vi "tmp-valveControl.vi"() -> ()   [LabVIEW 2016]
uses:
  Classes/Controllers/I-O/Copy of NI-DAQ Folder/NI-DAQ.lvclass
panel:
  in  "values":bool[](array[boolean])=[TRUE]
  in  "indices":i32[](array[numeric])=[0]
  in  "DAQ Module":i32
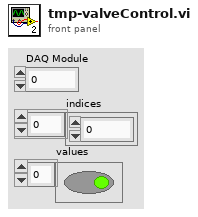
[diagram p1: front panel]
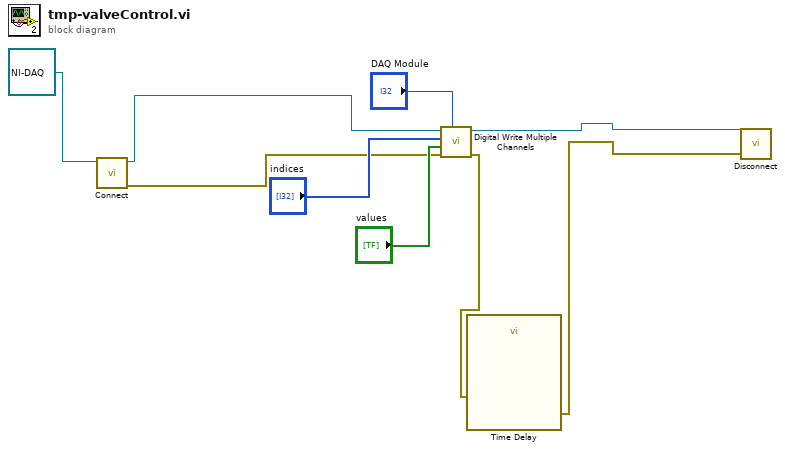
[diagram p0: block diagram]
diagram:
  n1 = call-dynamic "Connect.vi"("NI-DAQ in"=refnum<class "NI-DAQ.lvclass"> refnum ("NI-DAQ.lvclass")) -> ("error out"=w4:errorcluster, "NI-DAQ out"=w5:refnum<class "NI-DAQ.lvclass">)  [unwired: 9 in]
  n2 = call-dynamic "Digital Write Multiple Channels.vi"("DAQ Module"="DAQ Module", "error in (no error)"=w4, "Values"="values", "Indices"="indices", "NI-DAQ in"=w5) -> ("error out"=w6:errorcluster, "NI-DAQ out"=w2:refnum<class "NI-DAQ.lvclass">)  [unwired: 5 in]
  n3 = call "Time Delay"("error in (no error)"=w6) -> ("error out"=w1:errorcluster)  [unwired: 10 in]
  n4 = call-dynamic "Disconnect.vi"("error in (no error)"=w1, "I-O in"=w2) -> ()  [unwired: 8 in, 1 out]
